vi "GCSTranslator DLL Functions.vi"(0 "System no.":i32=1 min=1 step=1, 1 "Function":T1(ring), 4 "String input":string, 5 "error in":errorcluster, 6 "String buffer":string, 7 "Numerical input":i32, 8 "String input 2":string) -> (14 "DLL I32 Return value":i32, 15 "Boolean output":bool, 16 "String output":string, 17 "Numerical output":i32, 19 "error out":errorcluster)   [LabVIEW 2020]
doc: "This VI calls a given function from GCSTranslator.dll. GCSTranslator.dll must be installed. To call a system-specific function, the system-specific GCS DLL must be installed also. \n\nWarning: For XXX_GcsGetANswer , String buffer must be large enough, otherwise the application may crash. Call XXX_GcsGetANswerSize first to determine necessary string length."
uses:
  Global1.vi
  Global DaisyChain.vi
panel:
  # "This vi calls a given function from GCSTranslator.dll. GCSTranslator.dll must be installed. \nThe system specific GCS DLL must be installed also.\nWARNING: For \"XXXX_GcsGetAnswer\" \"String buffer\" must be large enough, otherwise the \napplication may crash. Call \"XXXX_GcsGetAnswerSize\" first to determine necessary string length."
  # "General inputs:"
  # "Function specific inputs:"
  # "Error handling:"
  # "DLL outputs:"
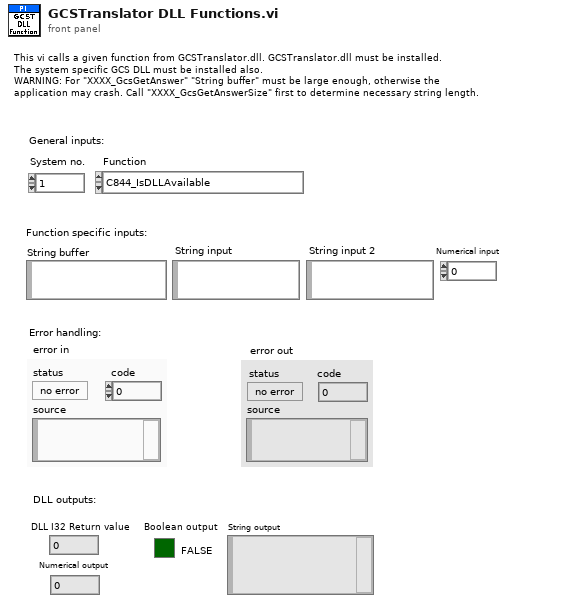
[diagram p1: front panel]
types:
  T1 = enum16{"C844_IsDLLAvailable", "C844_ConnectRS232", "C844_ConnectNIgpib", "C844_IsConnected", "C844_CloseConnection", "C844_GcsCommandset", "C844_GetError", "C844_GcsGetAnswerSize", "C844_GcsGetAnswer", "C843_IsDLLAvailable", "C843_Connect", "C843_IsConnected", "C843_CloseConnection", "C843_GcsCommandset", "C843_GetError", "C843_GcsGetAnswerSize", "C843_GcsGetAnswer", "E710_IsDLLAvailable", "E710_ConnectRS232", "E710_ConnectNIgpib", "E710_IsConnected", "E710_CloseConnection", "E710_GcsCommandset", "E710_GetError", "E710_GcsGetAnswerSize", "E710_GcsGetAnswer", "C843_PM_IsDLLAvailable", "C843_PM_Connect", "C843_PM_IsConnected", "C843_PM_CloseConnection", "C843_PM_GcsCommandset", "C843_PM_GetError", "C843_PM_GcsGetAnswerSize", "C843_PM_GcsGetAnswer", "C843_PM_GetCurrentBoardID", "C843_GetCurrentBoardID", "C865_IsDLLAvailable", "C865_ConnectRS232", "C865_IsConnected", "C865_CloseConnection", "C865_GcsCommandset", "C865_GetError", "C865_GcsGetAnswerSize", "C865_GcsGetAnswer", "C865_GetCurrentInterfaceID", "E761_ConnectPciBoard", "DefineSystem", "CloseConnection", "IsConnected", "ConnectRS232", "ConnectNIgpib", "ConnectPciBoard", "ConnectTCPIP", "GetError", "GcsCommandset", "GCSGetAnswerSize", "GcsGetAnswer", "CloseDaisyChain", "OpenRS232DaisyChain", "ConnectDaisyChainDevice", "ConnectUSB", "ListUSB", "OpenUSBDaisyChain", "OpenTCPIPDaisyChain"}
  T2 = typedef "Available interfaces.ctl" = u16
  T3 = cluster{"RS232 Portnumber":i32, "Timeout":i32, "RS232 Baud rate":u32, "Interface":T2, "GPIB Bus":i32, "GPIB Address":i32, "GPIB Mode":i32}[]
  T4 = cluster{"RS232 Portnumber":i32, "Timeout":i32, "RS232 Baud rate":u32, "Interface":T2, "GPIB Bus":i32, "GPIB Address":i32, "GPIB Mode":i32}
  T5 = typedef "Available DLLs.ctl" = u16
  T6 = typedef "Available DLL interfaces.ctl" = u16
  T7 = cluster{"DLL for Device":T5, "DLL Interface":T6, "Parameter":string}[]
  T8 = cluster{"DLL for Device":T5, "DLL Interface":T6, "Parameter":string}
  T9 = cluster{"No. of devices":i32, "Port ID":i32, "Devices":string[], "Description":string}[]
  T10 = cluster{"No. of devices":i32, "Port ID":i32, "Devices":string[], "Description":string}
  T11 = cluster{"Host address/name":string, "Port":i32, "Board":i32}[]
  T12 = cluster{"Host address/name":string, "Port":i32, "Board":i32}
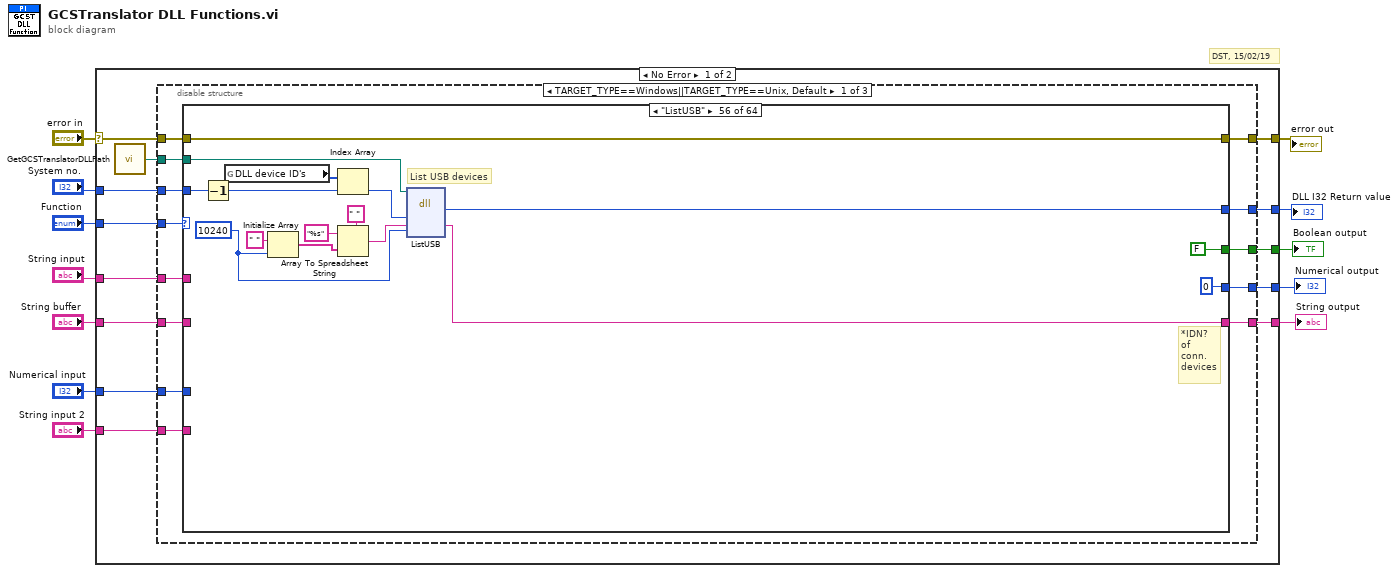
[diagram p0: block diagram]
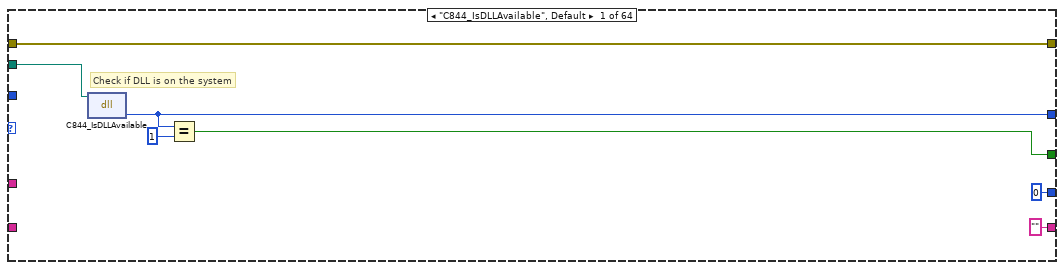
[diagram p2: hidden frame]
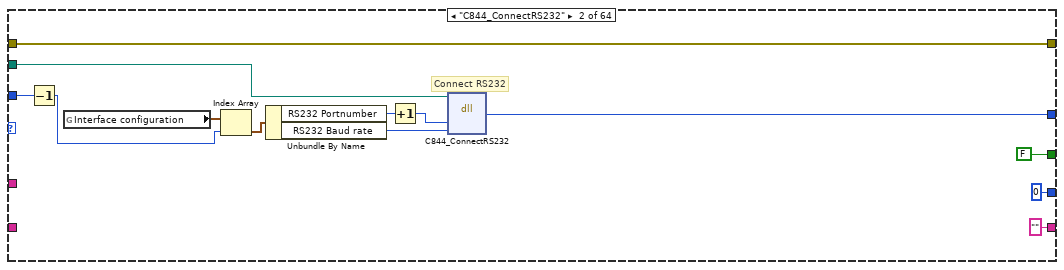
[diagram p3: hidden frame]
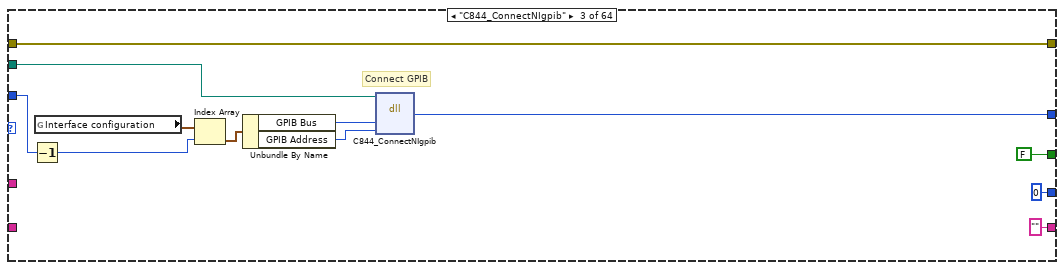
[diagram p4: hidden frame]
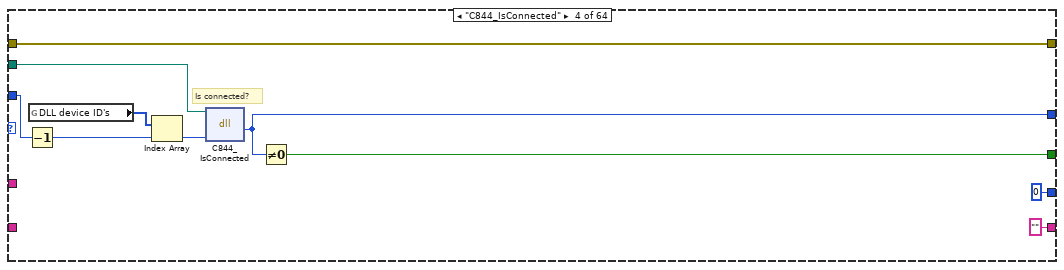
[diagram p5: hidden frame]
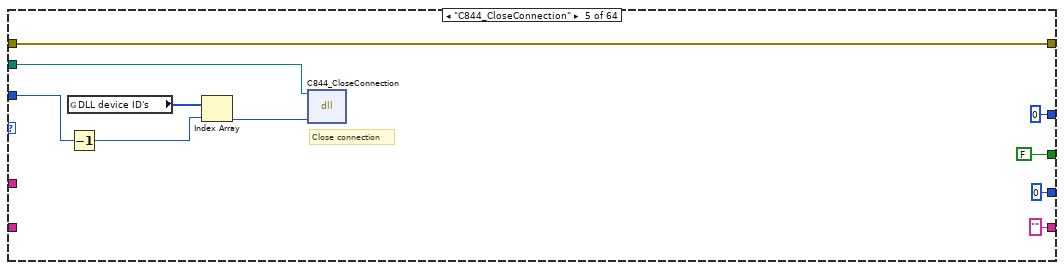
[diagram p6: hidden frame]
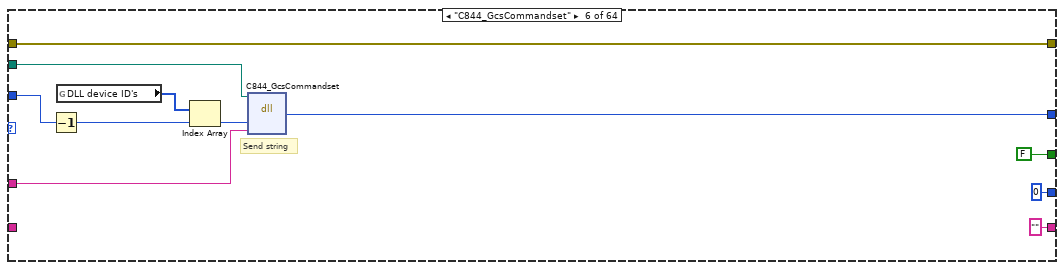
[diagram p7: hidden frame]
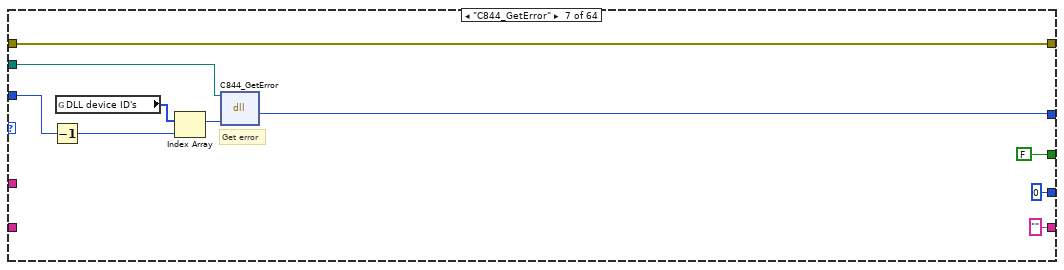
[diagram p8: hidden frame]
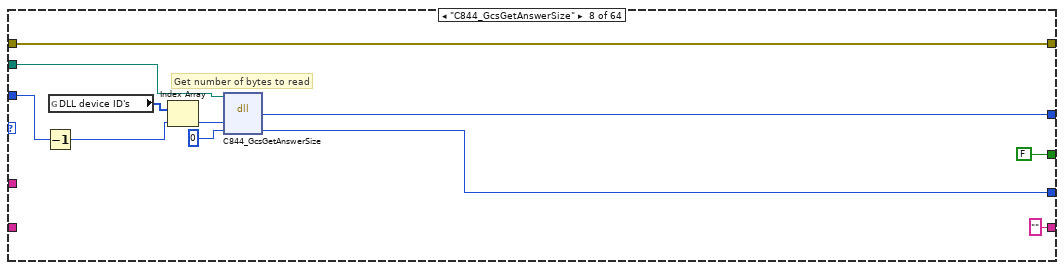
[diagram p9: hidden frame]
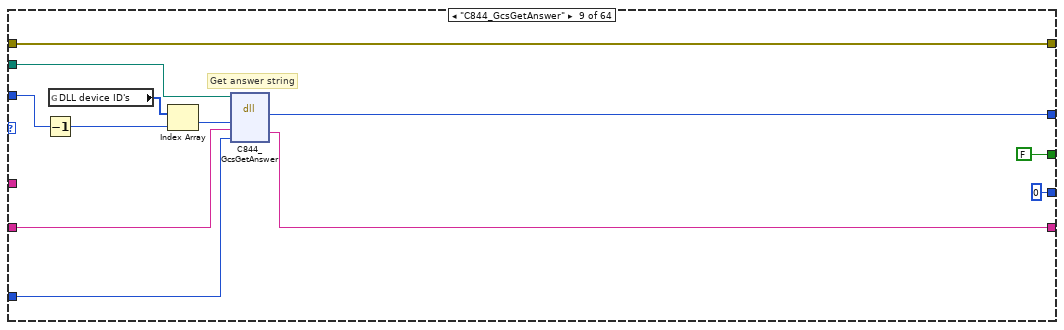
[diagram p10: hidden frame]
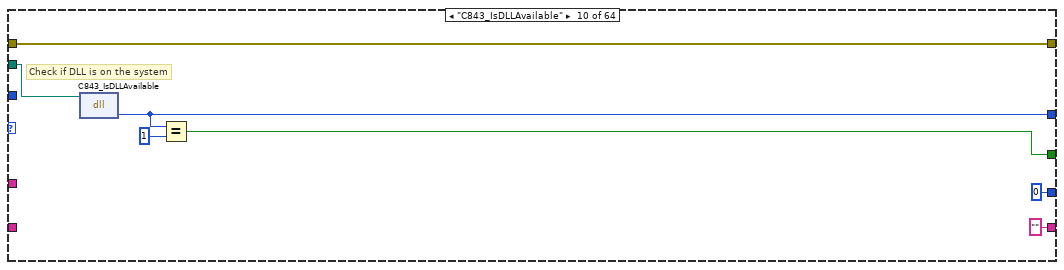
[diagram p11: hidden frame]
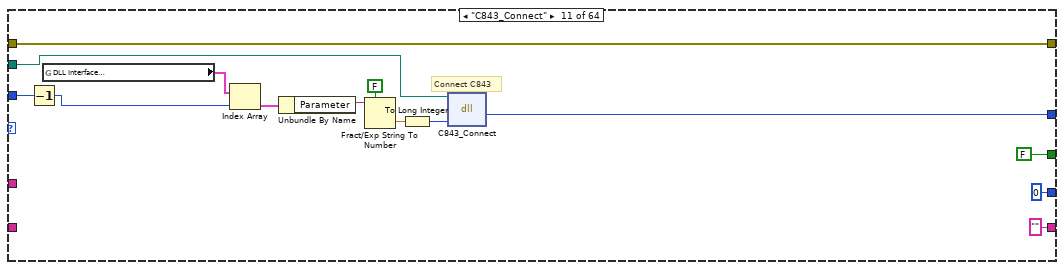
[diagram p12: hidden frame]
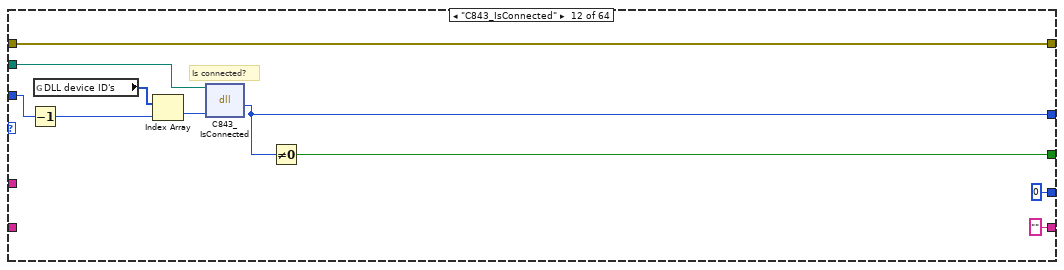
[diagram p13: hidden frame]
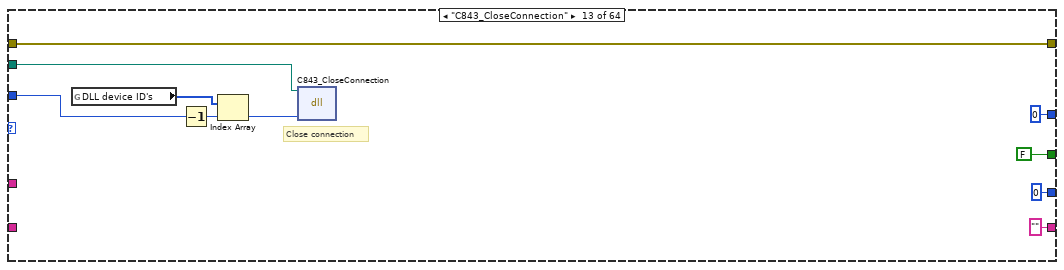
[diagram p14: hidden frame]
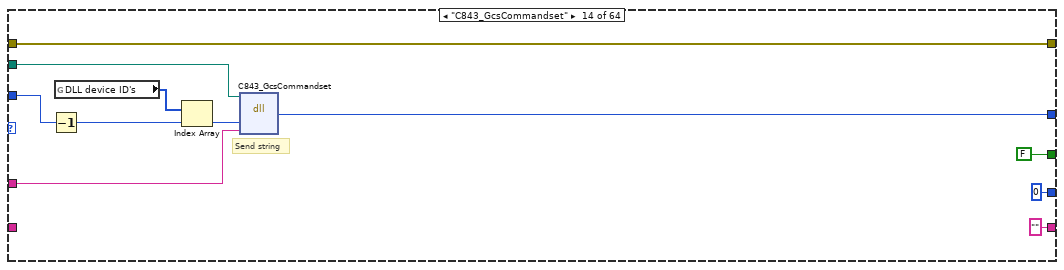
[diagram p15: hidden frame]
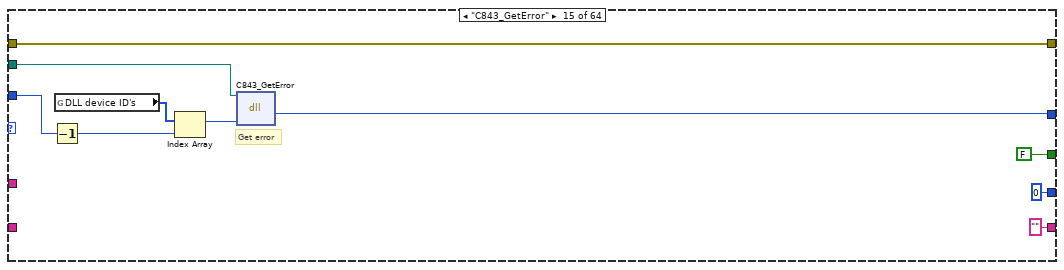
[diagram p16: hidden frame]
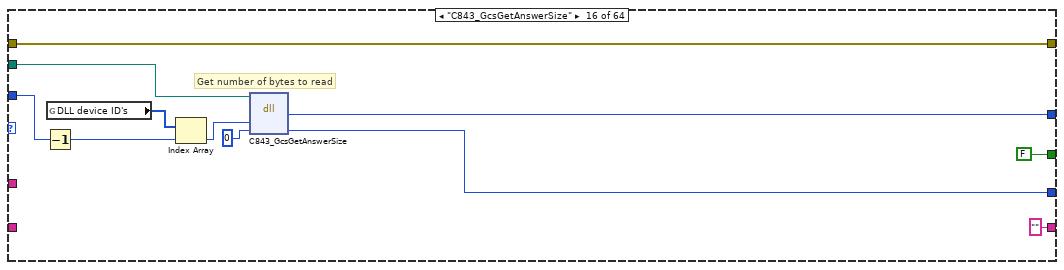
[diagram p17: hidden frame]
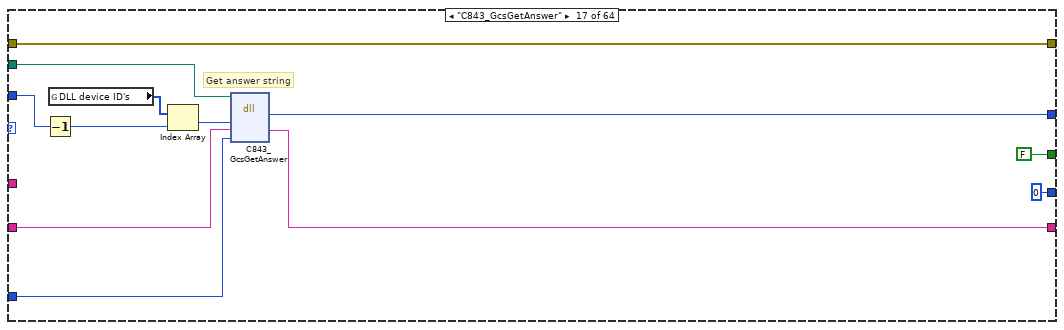
[diagram p18: hidden frame]
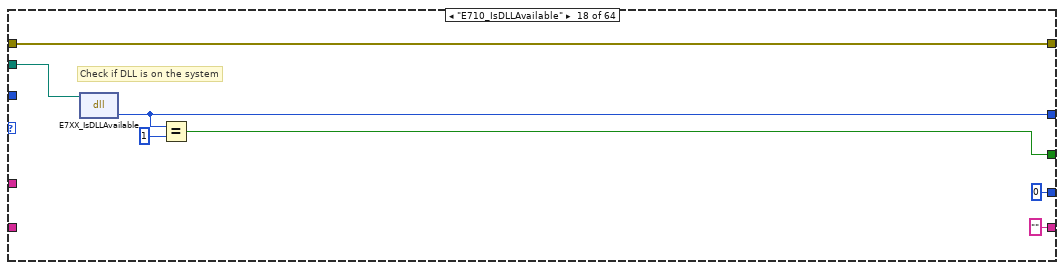
[diagram p19: hidden frame]
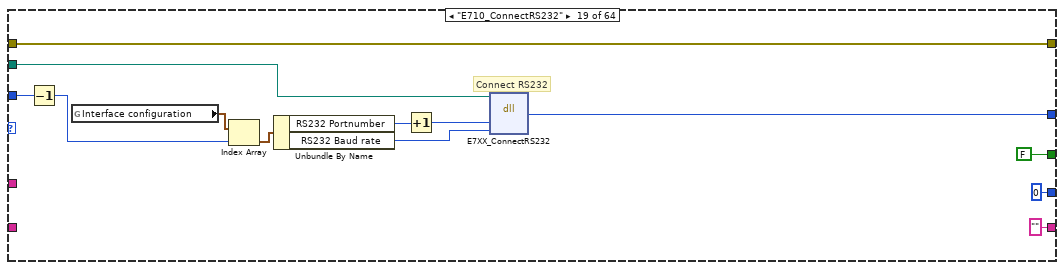
[diagram p20: hidden frame]
diagram:
  # "DST, 15/02/19"
  n1 = case shown="No Error" "error in" {
    selector: "error in" -> [w16 w891]
    tunnel: [w25 w891] -> w12
    tunnel: [w24 0] -> w11
    tunnel: [w23 FALSE] -> w10
    tunnel: "String input" -> [w22 _]
    tunnel: [w21 0 ("iAnswerSize")] -> w8
    tunnel: "String buffer" -> [w20 _]
    tunnel: [w19 "" ("szAnswer")] -> w6
    tunnel: "Numerical input" -> [w18 _]
    tunnel: "String input 2" -> [w17 _]
    tunnel: "System no." -> [w15 _]
    tunnel: "Function" -> [w14 _]
    frame No Error {
      n2 = call "GetGCSTranslatorDLLPath.vi"() -> ("DLL path"=w13:path)  [unwired: 1 in]
      n3 = disable-structure shown="TARGET_TYPE==Windows||TARGET_TYPE==Unix, Default" {
        disable-tunnel: w14 -> [w38 _ _]
        disable-tunnel: w16 -> [w37 w889 w890]
        disable-tunnel: [w36 w889 w890] -> w25
        disable-tunnel: [w35 _ _] -> w24
        disable-tunnel: w15 -> [w34 _ _]
        disable-tunnel: [w33 _ _] -> w23
        disable-tunnel: w22 -> [w32 _ _]
        disable-tunnel: [w31 _ _] -> w21
        disable-tunnel: w20 -> [w30 _ _]
        disable-tunnel: [w29 _ _] -> w19
        disable-tunnel: w18 -> [w28 _ _]
        disable-tunnel: w17 -> [w27 _ _]
        disable-tunnel: w13 -> [w26 _ _]
        frame condition #0 (active) {
          n4 = case shown="\"ListUSB\"" w38 {
            tunnel: w34 -> [_ w52 w65 w75 w85 w96 w106 w116 w129 _ w152 w160 w170 w181 w191 w201 w214 _ w233 w246 w256 w266 w277 w287 w297 w310 _ w334 w341 w351 w362 w372 w382 w395 w411 w425 _ w443 w453 w463 w474 w484 w494 w507 w523 _ w539 w547 w582 w599 w621 w650 w700 w733 w762 w778 w790 w806 w820 w834 w845 w860 w870 w883]
            tunnel: w37 -> [w45 w50 w63 w78 w90 w101 w111 w122 w134 w141 w150 w163 w175 w186 w196 w207 w219 w226 w231 w244 w259 w271 w282 w292 w303 w315 w322 w332 w344 w356 w367 w377 w388 w400 w409 w423 w435 w441 w456 w468 w479 w489 w500 w512 w521 w531 w544 w560 w585 w597 w607 w641 w699 w732 w761 w777 w788 w804 w818 w833 w840 w865 w876 w888]
            tunnel: [w45 w50 w63 w78 w90 w101 w111 w122 w134 w141 w150 w163 w175 w186 w196 w207 w219 w226 w231 w244 w259 w271 w282 w292 w303 w315 w322 w332 w344 w356 w367 w377 w388 w400 w409 w423 w435 w441 w456 w468 w479 w489 w500 w512 w521 w531 w544 w560 w585 w597 w606 w640 w699 w732 w761 w777 w788 w804 w818 w833 w839 w865 w876 w888] -> w36
            tunnel: [w44 w51 w64 w77 0 w100 w110 w120 w133 w140 w151 w162 0 w185 w195 w205 w218 w225 w232 w245 w258 0 w281 w291 w301 w314 w321 w333 w343 0 w366 w376 w386 w399 w410 w424 w434 w442 w455 0 w478 w488 w498 w511 w522 w532 0 0 w584 w598 w620 w649 w676 w715 w750 w768 w789 w805 w819 w827 w838 w864 w874 w887] -> w35
            tunnel: [w42 FALSE FALSE w74 FALSE FALSE FALSE FALSE FALSE w138 FALSE w159 FALSE FALSE FALSE FALSE FALSE w223 FALSE FALSE w255 FALSE FALSE FALSE FALSE FALSE w319 FALSE w340 FALSE FALSE FALSE FALSE FALSE FALSE FALSE w432 FALSE w452 FALSE FALSE FALSE FALSE FALSE FALSE FALSE FALSE FALSE w581 FALSE FALSE FALSE FALSE FALSE FALSE FALSE FALSE FALSE FALSE FALSE FALSE FALSE FALSE FALSE] -> w33
            tunnel: w32 -> [_ _ _ _ _ w94 _ _ _ _ _ _ _ w179 _ _ _ _ _ _ _ _ w275 _ _ _ _ _ _ _ w360 _ _ _ _ _ _ _ _ _ w472 _ _ _ _ w534 _ _ _ _ _ _ _ _ _ _ _ _ _ _ _ w858 _ _]
            tunnel: [0 ("iAnswerSize") 0 ("iAnswerSize") 0 ("iAnswerSize") 0 ("iAnswerSize") 0 ("iAnswerSize") 0 ("iAnswerSize") 0 ("iAnswerSize") w114 0 ("iAnswerSize") 0 ("iAnswerSize") 0 ("iAnswerSize") 0 ("iAnswerSize") 0 ("iAnswerSize") 0 ("iAnswerSize") 0 ("iAnswerSize") w199 0 ("iAnswerSize") 0 ("iAnswerSize") 0 ("iAnswerSize") 0 ("iAnswerSize") 0 ("iAnswerSize") 0 ("iAnswerSize") 0 ("iAnswerSize") 0 ("iAnswerSize") w295 0 ("iAnswerSize") 0 ("iAnswerSize") 0 ("iAnswerSize") 0 ("iAnswerSize") 0 ("iAnswerSize") 0 ("iAnswerSize") 0 ("iAnswerSize") w380 0 ("iAnswerSize") 0 ("iAnswerSize") 0 ("iAnswerSize") 0 ("iAnswerSize") 0 ("iAnswerSize") 0 ("iAnswerSize") 0 ("iAnswerSize") 0 ("iAnswerSize") 0 ("iAnswerSize") w492 0 ("iAnswerSize") 0 ("iAnswerSize") 0 ("iAnswerSize") 0 ("iAnswerSize") 0 ("iAnswerSize") 0 ("iAnswerSize") 0 ("iAnswerSize") 0 ("iAnswerSize") 0 ("iAnswerSize") w675 w714 w747 0 ("iAnswerSize") 0 ("iAnswerSize") 0 ("iAnswerSize") 0 ("iAnswerSize") 0 ("iAnswerSize") 0 ("iAnswerSize") 0 ("iAnswerSize") w868 0 ("iAnswerSize")] -> w31
            tunnel: w30 -> [_ _ _ _ _ _ _ _ w127 _ _ _ _ _ _ _ w212 _ _ _ _ _ _ _ _ w308 _ _ _ _ _ _ _ w393 _ _ _ _ _ _ _ _ _ w505 _ _ _ _ _ _ _ _ _ _ _ _ _ _ _ _ _ _ _ w881]
            tunnel: ["" ("szAnswer") "" ("szAnswer") "" ("szAnswer") "" ("szAnswer") "" ("szAnswer") "" ("szAnswer") "" ("szAnswer") "" ("szAnswer") w126 "" ("szAnswer") "" ("szAnswer") "" ("szAnswer") "" ("szAnswer") "" ("szAnswer") "" ("szAnswer") "" ("szAnswer") w211 "" ("szAnswer") "" ("szAnswer") "" ("szAnswer") "" ("szAnswer") "" ("szAnswer") "" ("szAnswer") "" ("szAnswer") "" ("szAnswer") w307 "" ("szAnswer") "" ("szAnswer") "" ("szAnswer") "" ("szAnswer") "" ("szAnswer") "" ("szAnswer") "" ("szAnswer") w392 "" ("szAnswer") "" ("szAnswer") "" ("szAnswer") "" ("szAnswer") "" ("szAnswer") "" ("szAnswer") "" ("szAnswer") "" ("szAnswer") "" ("szAnswer") w504 "" ("szAnswer") "" ("szAnswer") "" ("szAnswer") "" ("szAnswer") "" ("szAnswer") "" ("szAnswer") "" ("szAnswer") "" ("szAnswer") w674 w713 w745 w766 "" ("szAnswer") "" ("szAnswer") "" ("szAnswer") "" ("szAnswer") "" ("szAnswer") "" ("szAnswer") "" ("szAnswer") w880] -> w29
            tunnel: w28 -> [_ _ _ _ _ _ _ _ w124 _ _ _ _ _ _ _ w209 _ _ _ _ _ _ _ _ w305 _ _ _ _ _ _ _ w390 _ _ _ _ _ _ _ _ _ w502 _ _ _ _ _ _ _ _ _ _ _ _ _ _ _ _ _ _ _ w878]
            tunnel: w27 -> [_ _ _ _ _ _ _ _ _ _ _ _ _ _ _ _ _ _ _ _ _ _ _ _ _ _ _ _ _ _ _ _ _ _ _ _ _ _ _ _ _ _ _ _ _ w533 _ _ _ _ _ _ _ _ _ _ _ _ _ _ _ _ _ _]
            tunnel: w26 -> [w39 w46 w59 w71 w81 w91 w102 w112 w123 w135 w142 w156 w166 w176 w187 w197 w208 w220 w227 w240 w252 w262 w272 w283 w293 w304 w316 w323 w337 w347 w357 w368 w378 w389 w401 w415 w429 w436 w449 w459 w469 w480 w490 w501 w513 w527 w535 w545 w578 w588 w603 w630 w665 w704 w736 w763 w779 w793 w809 w823 w837 w855 w866 w877]
            frame "C844_IsDLLAvailable", Default {
              # "Check if DLL is on the system"
              n5 = dll-call lib="T:/Entwicklung/HostSoftware/LabVIEW/GCSDrivers/source/GCS2LabVIEW/Low Level/GCSTranslator.dll" fn="C844_IsDLLAvailable"(path in=w39) -> ("return type"=w44:i32)  [unwired: 2 in, 2 out]
              n6 = Equal?(x=w44, y=1) -> (x = y?=w42:bool)
            }
            frame "C844_ConnectRS232" {
              # "Connect RS232"
              n7 = Decrement(x=w52) -> (x-1=w54:i32)
              n8 = global read "Global1.vi" "Interface configuration"() -> (w55:T3)
              n9 = Index Array(array=w55, index=w54) -> (element=w53:T4)
              n10 = Unbundle By Name(w53) -> ("RS232 Portnumber"=w56:i32, "RS232 Baud rate"=w58:u32)
              n11 = Increment(x=w56) -> (x+1=w57:i32)
              n12 = dll-call lib="T:/Entwicklung/HostSoftware/LabVIEW/GCSDrivers/source/GCS2LabVIEW/Low Level/GCSTranslator.dll" fn="C844_ConnectRS232"(path in=w46, "nPortNr"=w57, "nBaudRate"=w58) -> ("return type"=w51:i32)  [unwired: 4 in, 2 out]
            }
            frame "C844_ConnectNIgpib" {
              # "Connect GPIB"
              n13 = Decrement(x=w65) -> (x-1=w67:i32)
              n14 = global read "Global1.vi" "Interface configuration"() -> (w68:T3)
              n15 = Index Array(array=w68, index=w67) -> (element=w66:T4)
              n16 = Unbundle By Name(w66) -> ("GPIB Bus"=w70:i32, "GPIB Address"=w69:i32)
              n17 = dll-call lib="T:/Entwicklung/HostSoftware/LabVIEW/GCSDrivers/source/GCS2LabVIEW/Low Level/GCSTranslator.dll" fn="C844_ConnectNIgpib"(path in=w59, "nBoard"=w70, "nDevAddr"=w69) -> ("return type"=w64:i32)  [unwired: 4 in, 2 out]
            }
            frame "C844_IsConnected" {
              # "Is connected?"
              n18 = Decrement(x=w75) -> (x-1=w79:i32)
              n19 = global read "Global1.vi" "DLL device ID's"() -> (w76:i32[])
              n20 = Index Array(array=w76, index=w79) -> (element=w80:i32)
              n21 = dll-call lib="T:/Entwicklung/HostSoftware/LabVIEW/GCSDrivers/source/GCS2LabVIEW/Low Level/GCSTranslator.dll" fn="C844_IsConnected"(path in=w71, "ID"=w80) -> ("return type"=w77:i32)  [unwired: 3 in, 2 out]
              n22 = Not Equal To 0?(x=w77) -> (x != 0?=w74:bool)
            }
            frame "C844_CloseConnection" {
              # "Close connection"
              n23 = global read "Global1.vi" "DLL device ID's"() -> (w87:i32[])
              n24 = Decrement(x=w85) -> (x-1=w88:i32)
              n25 = Index Array(array=w87, index=w88) -> (element=w86:i32)
              n26 = dll-call lib="T:/Entwicklung/HostSoftware/LabVIEW/GCSDrivers/source/GCS2LabVIEW/Low Level/GCSTranslator.dll" fn="C844_CloseConnection"(path in=w81, "ID"=w86) -> ()  [unwired: 3 in, 3 out]
            }
            frame "C844_GcsCommandset" {
              # "Send string"
              n27 = Decrement(x=w96) -> (x-1=w99:i32)
              n28 = global read "Global1.vi" "DLL device ID's"() -> (w98:i32[])
              n29 = Index Array(array=w98, index=w99) -> (element=w97:i32)
              n30 = dll-call lib="T:/Entwicklung/HostSoftware/LabVIEW/GCSDrivers/source/GCS2LabVIEW/Low Level/GCSTranslator.dll" fn="C844_GcsCommandset"(path in=w91, "ID"=w97, "szCommand"=w94) -> ("return type"=w100:i32)  [unwired: 4 in, 2 out]
            }
            frame "C844_GetError" {
              # "Get error"
              n31 = Decrement(x=w106) -> (x-1=w109:i32)
              n32 = global read "Global1.vi" "DLL device ID's"() -> (w108:i32[])
              n33 = Index Array(array=w108, index=w109) -> (element=w107:i32)
              n34 = dll-call lib="T:/Entwicklung/HostSoftware/LabVIEW/GCSDrivers/source/GCS2LabVIEW/Low Level/GCSTranslator.dll" fn="C844_GetError"(path in=w102, "ID"=w107) -> ("return type"=w110:i32)  [unwired: 3 in, 2 out]
            }
            frame "C844_GcsGetAnswerSize" {
              # "Get number of bytes to read"
              n35 = Decrement(x=w116) -> (x-1=w119:i32)
              n36 = global read "Global1.vi" "DLL device ID's"() -> (w118:i32[])
              n37 = Index Array(array=w118, index=w119) -> (element=w117:i32)
              n38 = dll-call lib="T:/Entwicklung/HostSoftware/LabVIEW/GCSDrivers/source/GCS2LabVIEW/Low Level/GCSTranslator.dll" fn="C844_GcsGetAnswerSize"(path in=w112, "ID"=w117, "iAnswerSize"=0) -> ("return type"=w120:i32, "iAnswerSize"=w114:i32)  [unwired: 3 in, 2 out]
            }
            frame "C844_GcsGetAnswer" {
              # "Get answer string"
              n39 = Decrement(x=w129) -> (x-1=w132:i32)
              n40 = global read "Global1.vi" "DLL device ID's"() -> (w131:i32[])
              n41 = Index Array(array=w131, index=w132) -> (element=w130:i32)
              n42 = dll-call lib="T:/Entwicklung/HostSoftware/LabVIEW/GCSDrivers/source/GCS2LabVIEW/Low Level/GCSTranslator.dll" fn="C844_GcsGetAnswer"(path in=w123, "ID"=w130, "szAnswer"=w127, "iAnswerSize"=w124) -> ("return type"=w133:i32, "szAnswer"=w126:string)  [unwired: 4 in, 2 out]
            }
            frame "C843_IsDLLAvailable" {
              # "Check if DLL is on the system"
              n43 = dll-call lib="T:/Entwicklung/HostSoftware/LabVIEW/GCSDrivers/source/GCS2LabVIEW/Low Level/GCSTranslator.dll" fn="C843_IsDLLAvailable"(path in=w135) -> ("return type"=w140:i32)  [unwired: 2 in, 2 out]
              n44 = Equal?(x=w140, y=1) -> (x = y?=w138:bool)
            }
            frame "C843_Connect" {
              # "Connect C843"
              n45 = Decrement(x=w152) -> (x-1=w154:i32)
              n46 = global read "Global1.vi" "DLL Interface\nConfiguration"() -> (w155:T7)
              n47 = Index Array(array=w155, index=w154) -> (element=w153:T8)
              n48 = Unbundle By Name(w153) -> ("Parameter"=w146:string)
              n49 = Fract/Exp String To Number(use system decimal point (T)=FALSE, string=w146) -> (number=w147:dbl)  [unwired: 3 out]
              n50 = To Long Integer(number=w147) -> (32bit integer=w145:i32)
              n51 = dll-call lib="T:/Entwicklung/HostSoftware/LabVIEW/GCSDrivers/source/GCS2LabVIEW/Low Level/GCSTranslator.dll" fn="C843_Connect"(path in=w142, "iBoardNumber"=w145) -> ("return type"=w151:i32)  [unwired: 3 in, 2 out]
            }
            frame "C843_IsConnected" {
              # "Is connected?"
              n52 = Decrement(x=w160) -> (x-1=w164:i32)
              n53 = global read "Global1.vi" "DLL device ID's"() -> (w161:i32[])
              n54 = Index Array(array=w161, index=w164) -> (element=w165:i32)
              n55 = dll-call lib="T:/Entwicklung/HostSoftware/LabVIEW/GCSDrivers/source/GCS2LabVIEW/Low Level/GCSTranslator.dll" fn="C843_IsConnected"(path in=w156, "ID"=w165) -> ("return type"=w162:i32)  [unwired: 3 in, 2 out]
              n56 = Not Equal To 0?(x=w162) -> (x != 0?=w159:bool)
            }
            frame "C843_CloseConnection" {
              # "Close connection"
              n57 = global read "Global1.vi" "DLL device ID's"() -> (w172:i32[])
              n58 = Decrement(x=w170) -> (x-1=w173:i32)
              n59 = Index Array(array=w172, index=w173) -> (element=w171:i32)
              n60 = dll-call lib="T:/Entwicklung/HostSoftware/LabVIEW/GCSDrivers/source/GCS2LabVIEW/Low Level/GCSTranslator.dll" fn="C843_CloseConnection"(path in=w166, "ID"=w171) -> ()  [unwired: 3 in, 3 out]
            }
            frame "C843_GcsCommandset" {
              # "Send string"
              n61 = Decrement(x=w181) -> (x-1=w184:i32)
              n62 = global read "Global1.vi" "DLL device ID's"() -> (w183:i32[])
              n63 = Index Array(array=w183, index=w184) -> (element=w182:i32)
              n64 = dll-call lib="T:/Entwicklung/HostSoftware/LabVIEW/GCSDrivers/source/GCS2LabVIEW/Low Level/GCSTranslator.dll" fn="C843_GcsCommandset"(path in=w176, "ID"=w182, "szCommand"=w179) -> ("return type"=w185:i32)  [unwired: 4 in, 2 out]
            }
            frame "C843_GetError" {
              # "Get error"
              n65 = Decrement(x=w191) -> (x-1=w194:i32)
              n66 = global read "Global1.vi" "DLL device ID's"() -> (w193:i32[])
              n67 = Index Array(array=w193, index=w194) -> (element=w192:i32)
              n68 = dll-call lib="T:/Entwicklung/HostSoftware/LabVIEW/GCSDrivers/source/GCS2LabVIEW/Low Level/GCSTranslator.dll" fn="C843_GetError"(path in=w187, "ID"=w192) -> ("return type"=w195:i32)  [unwired: 3 in, 2 out]
            }
            frame "C843_GcsGetAnswerSize" {
              # "Get number of bytes to read"
              n69 = Decrement(x=w201) -> (x-1=w204:i32)
              n70 = global read "Global1.vi" "DLL device ID's"() -> (w203:i32[])
              n71 = Index Array(array=w203, index=w204) -> (element=w202:i32)
              n72 = dll-call lib="T:/Entwicklung/HostSoftware/LabVIEW/GCSDrivers/source/GCS2LabVIEW/Low Level/GCSTranslator.dll" fn="C843_GcsGetAnswerSize"(path in=w197, "ID"=w202, "iAnswerSize"=0) -> ("return type"=w205:i32, "iAnswerSize"=w199:i32)  [unwired: 3 in, 2 out]
            }
            frame "C843_GcsGetAnswer" {
              # "Get answer string"
              n73 = Decrement(x=w214) -> (x-1=w217:i32)
              n74 = global read "Global1.vi" "DLL device ID's"() -> (w216:i32[])
              n75 = Index Array(array=w216, index=w217) -> (element=w215:i32)
              n76 = dll-call lib="T:/Entwicklung/HostSoftware/LabVIEW/GCSDrivers/source/GCS2LabVIEW/Low Level/GCSTranslator.dll" fn="C843_GcsGetAnswer"(path in=w208, "ID"=w215, "szAnswer"=w212, "iAnswerSize"=w209) -> ("return type"=w218:i32, "szAnswer"=w211:string)  [unwired: 4 in, 2 out]
            }
            frame "E710_IsDLLAvailable" {
              # "Check if DLL is on the system"
              n77 = dll-call lib="T:/Entwicklung/HostSoftware/LabVIEW/GCSDrivers/source/GCS2LabVIEW/Low Level/GCSTranslator.dll" fn="E7XX_IsDLLAvailable"(path in=w220) -> ("return type"=w225:i32)  [unwired: 2 in, 2 out]
              n78 = Equal?(x=w225, y=1) -> (x = y?=w223:bool)
            }
            frame "E710_ConnectRS232" {
              # "Connect RS232"
              n79 = Decrement(x=w233) -> (x-1=w235:i32)
              n80 = global read "Global1.vi" "Interface configuration"() -> (w236:T3)
              n81 = Index Array(array=w236, index=w235) -> (element=w234:T4)
              n82 = Unbundle By Name(w234) -> ("RS232 Portnumber"=w237:i32, "RS232 Baud rate"=w239:u32)
              n83 = Increment(x=w237) -> (x+1=w238:i32)
              n84 = dll-call lib="T:/Entwicklung/HostSoftware/LabVIEW/GCSDrivers/source/GCS2LabVIEW/Low Level/GCSTranslator.dll" fn="E7XX_ConnectRS232"(path in=w227, "nPortNr"=w238, "nBaudRate"=w239) -> ("return type"=w232:i32)  [unwired: 4 in, 2 out]
            }
            frame "E710_ConnectNIgpib" {
              # "Connect GPIB"
              n85 = Decrement(x=w246) -> (x-1=w248:i32)
              n86 = global read "Global1.vi" "Interface configuration"() -> (w249:T3)
              n87 = Index Array(array=w249, index=w248) -> (element=w247:T4)
              n88 = Unbundle By Name(w247) -> ("GPIB Bus"=w251:i32, "GPIB Address"=w250:i32)
              n89 = dll-call lib="T:/Entwicklung/HostSoftware/LabVIEW/GCSDrivers/source/GCS2LabVIEW/Low Level/GCSTranslator.dll" fn="E7XX_ConnectNIgpib"(path in=w240, "nBoard"=w251, "nDevAddr"=w250) -> ("return type"=w245:i32)  [unwired: 4 in, 2 out]
            }
            frame "E710_IsConnected" {
              # "Is connected?"
              n90 = global read "Global1.vi" "DLL device ID's"() -> (w257:i32[])
              n91 = Decrement(x=w256) -> (x-1=w260:i32)
              n92 = Index Array(array=w257, index=w260) -> (element=w261:i32)
              n93 = dll-call lib="T:/Entwicklung/HostSoftware/LabVIEW/GCSDrivers/source/GCS2LabVIEW/Low Level/GCSTranslator.dll" fn="E7XX_IsConnected"(path in=w252, "ID"=w261) -> ("return type"=w258:i32)  [unwired: 3 in, 2 out]
              n94 = Not Equal To 0?(x=w258) -> (x != 0?=w255:bool)
            }
            frame "E710_CloseConnection" {
              # "Close connection"
              n95 = global read "Global1.vi" "DLL device ID's"() -> (w268:i32[])
              n96 = Decrement(x=w266) -> (x-1=w269:i32)
              n97 = Index Array(array=w268, index=w269) -> (element=w267:i32)
              n98 = dll-call lib="T:/Entwicklung/HostSoftware/LabVIEW/GCSDrivers/source/GCS2LabVIEW/Low Level/GCSTranslator.dll" fn="E7XX_CloseConnection"(path in=w262, "ID"=w267) -> ()  [unwired: 3 in, 3 out]
            }
            frame "E710_GcsCommandset" {
              # "Send string"
              n99 = global read "Global1.vi" "DLL device ID's"() -> (w279:i32[])
              n100 = Decrement(x=w277) -> (x-1=w280:i32)
              n101 = Index Array(array=w279, index=w280) -> (element=w278:i32)
              n102 = dll-call lib="T:/Entwicklung/HostSoftware/LabVIEW/GCSDrivers/source/GCS2LabVIEW/Low Level/GCSTranslator.dll" fn="E7XX_GcsCommandset"(path in=w272, "ID"=w278, "szCommand"=w275) -> ("return type"=w281:i32)  [unwired: 4 in, 2 out]
            }
            frame "E710_GetError" {
              # "Get error"
              n103 = Decrement(x=w287) -> (x-1=w290:i32)
              n104 = global read "Global1.vi" "DLL device ID's"() -> (w289:i32[])
              n105 = Index Array(array=w289, index=w290) -> (element=w288:i32)
              n106 = dll-call lib="T:/Entwicklung/HostSoftware/LabVIEW/GCSDrivers/source/GCS2LabVIEW/Low Level/GCSTranslator.dll" fn="E7XX_GetError"(path in=w283, "ID"=w288) -> ("return type"=w291:i32)  [unwired: 3 in, 2 out]
            }
            frame "E710_GcsGetAnswerSize" {
              # "Get number of bytes to read"
              n107 = Decrement(x=w297) -> (x-1=w300:i32)
              n108 = global read "Global1.vi" "DLL device ID's"() -> (w299:i32[])
              n109 = Index Array(array=w299, index=w300) -> (element=w298:i32)
              n110 = dll-call lib="T:/Entwicklung/HostSoftware/LabVIEW/GCSDrivers/source/GCS2LabVIEW/Low Level/GCSTranslator.dll" fn="E7XX_GcsGetAnswerSize"(path in=w293, "ID"=w298, "iAnswerSize"=0) -> ("return type"=w301:i32, "iAnswerSize"=w295:i32)  [unwired: 3 in, 2 out]
            }
            frame "E710_GcsGetAnswer" {
              # "Get answer string"
              n111 = Decrement(x=w310) -> (x-1=w313:i32)
              n112 = global read "Global1.vi" "DLL device ID's"() -> (w312:i32[])
              n113 = Index Array(array=w312, index=w313) -> (element=w311:i32)
              n114 = dll-call lib="T:/Entwicklung/HostSoftware/LabVIEW/GCSDrivers/source/GCS2LabVIEW/Low Level/GCSTranslator.dll" fn="E7XX_GcsGetAnswer"(path in=w304, "ID"=w311, "szAnswer"=w308, "iAnswerSize"=w305) -> ("return type"=w314:i32, "szAnswer"=w307:string)  [unwired: 4 in, 2 out]
            }
            frame "C843_PM_IsDLLAvailable" {
              # "Check if DLL is on the system"
              n115 = dll-call lib="T:/Entwicklung/HostSoftware/LabVIEW/GCSDrivers/source/GCS2LabVIEW/Low Level/GCSTranslator.dll" fn="C843_PM_IsDLLAvailable"(path in=w316) -> ("return type"=w321:i32)  [unwired: 2 in, 2 out]
              n116 = Equal?(x=w321, y=1) -> (x = y?=w319:bool)
            }
            frame "C843_PM_Connect" {
              # "Connect C843_PM"
              n117 = Decrement(x=w334) -> (x-1=w324:i32)
              n118 = global read "Global1.vi" "DLL Interface\nConfiguration"() -> (w336:T7)
              n119 = Index Array(array=w336, index=w324) -> (element=w335:T8)
              n120 = Unbundle By Name(w335) -> ("Parameter"=w328:string)
              n121 = Fract/Exp String To Number(use system decimal point (T)=FALSE, string=w328) -> (number=w329:dbl)  [unwired: 3 out]
              n122 = To Long Integer(number=w329) -> (32bit integer=w327:i32)
              n123 = dll-call lib="T:/Entwicklung/HostSoftware/LabVIEW/GCSDrivers/source/GCS2LabVIEW/Low Level/GCSTranslator.dll" fn="C843_PM_Connect"(path in=w323, "iBoardNumber"=w327) -> ("return type"=w333:i32)  [unwired: 3 in, 2 out]
            }
            frame "C843_PM_IsConnected" {
              # "Is connected?"
              n124 = Decrement(x=w341) -> (x-1=w345:i32)
              n125 = global read "Global1.vi" "DLL device ID's"() -> (w342:i32[])
              n126 = Index Array(array=w342, index=w345) -> (element=w346:i32)
              n127 = dll-call lib="T:/Entwicklung/HostSoftware/LabVIEW/GCSDrivers/source/GCS2LabVIEW/Low Level/GCSTranslator.dll" fn="C843_PM_IsConnected"(path in=w337, "ID"=w346) -> ("return type"=w343:i32)  [unwired: 3 in, 2 out]
              n128 = Not Equal To 0?(x=w343) -> (x != 0?=w340:bool)
            }
            frame "C843_PM_CloseConnection" {
              # "Close connection"
              n129 = Decrement(x=w351) -> (x-1=w354:i32)
              n130 = global read "Global1.vi" "DLL device ID's"() -> (w353:i32[])
              n131 = Index Array(array=w353, index=w354) -> (element=w352:i32)
              n132 = dll-call lib="T:/Entwicklung/HostSoftware/LabVIEW/GCSDrivers/source/GCS2LabVIEW/Low Level/GCSTranslator.dll" fn="C843_PM_CloseConnection"(path in=w347, "ID"=w352) -> ()  [unwired: 3 in, 3 out]
            }
            frame "C843_PM_GcsCommandset" {
              # "Send string"
              n133 = Decrement(x=w362) -> (x-1=w365:i32)
              n134 = global read "Global1.vi" "DLL device ID's"() -> (w364:i32[])
              n135 = Index Array(array=w364, index=w365) -> (element=w363:i32)
              n136 = dll-call lib="T:/Entwicklung/HostSoftware/LabVIEW/GCSDrivers/source/GCS2LabVIEW/Low Level/GCSTranslator.dll" fn="C843_PM_GcsCommandset"(path in=w357, "ID"=w363, "szCommand"=w360) -> ("return type"=w366:i32)  [unwired: 4 in, 2 out]
            }
            frame "C843_PM_GetError" {
              # "Get error"
              n137 = Decrement(x=w372) -> (x-1=w375:i32)
              n138 = global read "Global1.vi" "DLL device ID's"() -> (w374:i32[])
              n139 = Index Array(array=w374, index=w375) -> (element=w373:i32)
              n140 = dll-call lib="T:/Entwicklung/HostSoftware/LabVIEW/GCSDrivers/source/GCS2LabVIEW/Low Level/GCSTranslator.dll" fn="C843_PM_GetError"(path in=w368, "ID"=w373) -> ("return type"=w376:i32)  [unwired: 3 in, 2 out]
            }
            frame "C843_PM_GcsGetAnswerSize" {
              # "Get number of bytes to read"
              n141 = Decrement(x=w382) -> (x-1=w385:i32)
              n142 = global read "Global1.vi" "DLL device ID's"() -> (w384:i32[])
              n143 = Index Array(array=w384, index=w385) -> (element=w383:i32)
              n144 = dll-call lib="T:/Entwicklung/HostSoftware/LabVIEW/GCSDrivers/source/GCS2LabVIEW/Low Level/GCSTranslator.dll" fn="C843_PM_GcsGetAnswerSize"(path in=w378, "ID"=w383, "iAnswerSize"=0) -> ("return type"=w386:i32, "iAnswerSize"=w380:i32)  [unwired: 3 in, 2 out]
            }
            frame "C843_PM_GcsGetAnswer" {
              # "Get answer string"
              n145 = Decrement(x=w395) -> (x-1=w398:i32)
              n146 = global read "Global1.vi" "DLL device ID's"() -> (w397:i32[])
              n147 = Index Array(array=w397, index=w398) -> (element=w396:i32)
              n148 = dll-call lib="T:/Entwicklung/HostSoftware/LabVIEW/GCSDrivers/source/GCS2LabVIEW/Low Level/GCSTranslator.dll" fn="C843_PM_GcsGetAnswer"(path in=w389, "ID"=w396, "szAnswer"=w393, "iAnswerSize"=w390) -> ("return type"=w399:i32, "szAnswer"=w392:string)  [unwired: 4 in, 2 out]
            }
            frame "C843_PM_GetCurrentBoardID" {
              # "Get current ID C843_PM"
              n149 = Decrement(x=w411) -> (x-1=w413:i32)
              n150 = global read "Global1.vi" "DLL Interface\nConfiguration"() -> (w414:T7)
              n151 = Index Array(array=w414, index=w413) -> (element=w412:T8)
              n152 = Unbundle By Name(w412) -> ("Parameter"=w405:string)
              n153 = Fract/Exp String To Number(use system decimal point (T)=FALSE, string=w405) -> (number=w406:dbl)  [unwired: 3 out]
              n154 = To Long Integer(number=w406) -> (32bit integer=w404:i32)
              n155 = dll-call lib="T:/Entwicklung/HostSoftware/LabVIEW/GCSDrivers/source/GCS2LabVIEW/Low Level/GCSTranslator.dll" fn="C843_PM_GetCurrentBoardId"(path in=w401, "iBoardNumber"=w404) -> ("return type"=w410:i32)  [unwired: 3 in, 2 out]
            }
            frame "C843_GetCurrentBoardID" {
              # "Get current ID C843"
              n156 = Decrement(x=w425) -> (x-1=w427:i32)
              n157 = global read "Global1.vi" "DLL Interface\nConfiguration"() -> (w428:T7)
              n158 = Index Array(array=w428, index=w427) -> (element=w426:T8)
              n159 = Unbundle By Name(w426) -> ("Parameter"=w419:string)
              n160 = Fract/Exp String To Number(use system decimal point (T)=FALSE, string=w419) -> (number=w420:dbl)  [unwired: 3 out]
              n161 = To Long Integer(number=w420) -> (32bit integer=w418:i32)
              n162 = dll-call lib="T:/Entwicklung/HostSoftware/LabVIEW/GCSDrivers/source/GCS2LabVIEW/Low Level/GCSTranslator.dll" fn="C843_GetCurrentBoardId"(path in=w415, "iBoardNumber"=w418) -> ("return type"=w424:i32)  [unwired: 3 in, 2 out]
            }
            frame "C865_IsDLLAvailable" {
              # "Check if DLL is on the system"
              n163 = dll-call lib="T:/Entwicklung/HostSoftware/LabVIEW/GCSDrivers/source/GCS2LabVIEW/Low Level/GCSTranslator.dll" fn="C865_IsDLLAvailable"(path in=w429) -> ("return type"=w434:i32)  [unwired: 2 in, 2 out]
              n164 = Equal?(x=w434, y=1) -> (x = y?=w432:bool)
            }
            frame "C865_ConnectRS232" {
              # "Connect RS232"
              n165 = Decrement(x=w443) -> (x-1=w437:i32)
              n166 = global read "Global1.vi" "Interface configuration"() -> (w445:T3)
              n167 = Index Array(array=w445, index=w437) -> (element=w444:T4)
              n168 = Unbundle By Name(w444) -> ("RS232 Portnumber"=w446:i32, "RS232 Baud rate"=w448:u32)
              n169 = Increment(x=w446) -> (x+1=w447:i32)
              n170 = dll-call lib="T:/Entwicklung/HostSoftware/LabVIEW/GCSDrivers/source/GCS2LabVIEW/Low Level/GCSTranslator.dll" fn="C865_ConnectRS232"(path in=w436, "nPortNr"=w447, "nBaudRate"=w448) -> ("return type"=w442:i32)  [unwired: 4 in, 2 out]
            }
            frame "C865_IsConnected" {
              # "Is connected?"
              n171 = global read "Global1.vi" "DLL device ID's"() -> (w454:i32[])
              n172 = Decrement(x=w453) -> (x-1=w457:i32)
              n173 = Index Array(array=w454, index=w457) -> (element=w458:i32)
              n174 = dll-call lib="T:/Entwicklung/HostSoftware/LabVIEW/GCSDrivers/source/GCS2LabVIEW/Low Level/GCSTranslator.dll" fn="C865_IsConnected"(path in=w449, "ID"=w458) -> ("return type"=w455:i32)  [unwired: 3 in, 2 out]
              n175 = Not Equal To 0?(x=w455) -> (x != 0?=w452:bool)
            }
            frame "C865_CloseConnection" {
              # "Close connection"
              n176 = global read "Global1.vi" "DLL device ID's"() -> (w465:i32[])
              n177 = Decrement(x=w463) -> (x-1=w466:i32)
              n178 = Index Array(array=w465, index=w466) -> (element=w464:i32)
              n179 = dll-call lib="T:/Entwicklung/HostSoftware/LabVIEW/GCSDrivers/source/GCS2LabVIEW/Low Level/GCSTranslator.dll" fn="C865_CloseConnection"(path in=w459, "ID"=w464) -> ()  [unwired: 3 in, 3 out]
            }
            frame "C865_GcsCommandset" {
              # "Send string"
              n180 = global read "Global1.vi" "DLL device ID's"() -> (w476:i32[])
              n181 = Decrement(x=w474) -> (x-1=w477:i32)
              n182 = Index Array(array=w476, index=w477) -> (element=w475:i32)
              n183 = dll-call lib="T:/Entwicklung/HostSoftware/LabVIEW/GCSDrivers/source/GCS2LabVIEW/Low Level/GCSTranslator.dll" fn="C865_GcsCommandset"(path in=w469, "ID"=w475, "szCommand"=w472) -> ("return type"=w478:i32)  [unwired: 4 in, 2 out]
            }
            frame "C865_GetError" {
              # "Get error"
              n184 = Decrement(x=w484) -> (x-1=w487:i32)
              n185 = global read "Global1.vi" "DLL device ID's"() -> (w486:i32[])
              n186 = Index Array(array=w486, index=w487) -> (element=w485:i32)
              n187 = dll-call lib="T:/Entwicklung/HostSoftware/LabVIEW/GCSDrivers/source/GCS2LabVIEW/Low Level/GCSTranslator.dll" fn="C865_GetError"(path in=w480, "ID"=w485) -> ("return type"=w488:i32)  [unwired: 3 in, 2 out]
            }
            frame "C865_GcsGetAnswerSize" {
              # "Get number of bytes to read"
              n188 = global read "Global1.vi" "DLL device ID's"() -> (w496:i32[])
              n189 = Decrement(x=w494) -> (x-1=w497:i32)
              n190 = Index Array(array=w496, index=w497) -> (element=w495:i32)
              n191 = dll-call lib="T:/Entwicklung/HostSoftware/LabVIEW/GCSDrivers/source/GCS2LabVIEW/Low Level/GCSTranslator.dll" fn="C865_GcsGetAnswerSize"(path in=w490, "ID"=w495, "iAnswerSize"=0) -> ("return type"=w498:i32, "iAnswerSize"=w492:i32)  [unwired: 3 in, 2 out]
            }
            frame "C865_GcsGetAnswer" {
              # "Get answer string"
              n192 = Decrement(x=w507) -> (x-1=w510:i32)
              n193 = global read "Global1.vi" "DLL device ID's"() -> (w509:i32[])
              n194 = Index Array(array=w509, index=w510) -> (element=w508:i32)
              n195 = dll-call lib="T:/Entwicklung/HostSoftware/LabVIEW/GCSDrivers/source/GCS2LabVIEW/Low Level/GCSTranslator.dll" fn="C865_GcsGetAnswer"(path in=w501, "ID"=w508, "szAnswer"=w505, "iAnswerSize"=w502) -> ("return type"=w511:i32, "szAnswer"=w504:string)  [unwired: 4 in, 2 out]
            }
            frame "C865_GetCurrentInterfaceID" {
              # "Get current ID C865"
              n196 = Decrement(x=w523) -> (x-1=w525:i32)
              n197 = global read "Global1.vi" "DLL Interface\nConfiguration"() -> (w526:T7)
              n198 = Index Array(array=w526, index=w525) -> (element=w524:T8)
              n199 = Unbundle By Name(w524) -> ("Parameter"=w517:string)
              n200 = Fract/Exp String To Number(use system decimal point (T)=FALSE, string=w517) -> (number=w518:dbl)  [unwired: 3 out]
              n201 = To Long Integer(number=w518) -> (32bit integer=w516:i32)
              n202 = dll-call lib="T:/Entwicklung/HostSoftware/LabVIEW/GCSDrivers/source/GCS2LabVIEW/Low Level/GCSTranslator.dll" fn="C865_GetCurrentInterfaceId"(path in=w513, "iBoardNumber"=w516) -> ("return type"=w522:i32)  [unwired: 3 in, 2 out]
            }
            frame "DefineSystem" {
              # "Define which GCS dll to use and for which system"
              n203 = dll-call lib="T:/Entwicklung/HostSoftware/LabVIEW/GCSDrivers/source/GCS2LabVIEW/Low Level/GCSTranslator.dll" fn="DefineSystem"(path in=w527, "szDLLName"=w534, "szCtrlPrefix"=w533) -> ("return type"=w532:i32)  [unwired: 4 in, 2 out]
            }
            frame "CloseConnection" {
              # "Close connection"
              n204 = global read "Global1.vi" "DLL device ID's"() -> (w541:i32[])
              n205 = Decrement(x=w539) -> (x-1=w542:i32)
              n206 = Index Array(array=w541, index=w542) -> (element=w540:i32)
              n207 = dll-call lib="T:/Entwicklung/HostSoftware/LabVIEW/GCSDrivers/source/GCS2LabVIEW/Low Level/GCSTranslator.dll" fn="CloseConnection"(path in=w535, "ID"=w540) -> ()  [unwired: 3 in, 3 out]
            }
            frame "CloseDaisyChain" {
              # "CloseDaisyChain"
              n208 = Decrement(x=w547) -> (x-1=w552:i32)
              n209 = global read "Global1.vi" "DLL device ID's"() -> (w558:i32[])
              n210 = global read "Global DaisyChain.vi" "DaisyChain configuration"() -> (w550:T9)
              n211 = global read "Global1.vi" "Number of\nsystems"() -> (w548:i32)
              n212 = Index Array(array=w558, index=w552) -> (element=w557:i32)
              n213 = Max & Min(x=w547, y=w548) -> (max(x,y)=w546:i32)  [unwired: 1 out]
              n214 = Index Array(array=w550, index=w552) -> (element=w553:T10)
              n215 = Unbundle By Name(w553) -> ("Port ID"=w551:i32)
              n216 = for {
                N: w546 -> [_]
                tunnel: w550 -> [w566]
                shift-right: [w568] -> w549
                shift-left: w550 -> [w567]
                tunnel: w551 -> [w564]
                i -> [w562]
                n217 = Index Array(array=w566, index=w562) -> (element=w561:T10)
                n218 = Unbundle By Name(w561) -> ("Port ID"=w565:i32)
                n219 = Equal?(x=w565, y=w564) -> (x = y?=w563:bool)
                n220 = case shown="True" w563 {
                  tunnel: [w569 w574] -> w568
                  tunnel: w567 -> [w569 w572]
                  tunnel: w562 -> [_ w573]
                  tunnel: w561 -> [_ w571]
                  frame False {
                  }
                  frame True {
                    n221 = Bundle By Name(cluster=w571, "Port ID"=-1, "No. of devices"=0, "Devices"=string[] []) -> (w570:T10)
                    n222 = Replace Array Subset(array=w572, new element=w570, index=w573) -> (w574:T9)
                  }
                }
              }
              n223 = dll-call lib="T:/Entwicklung/HostSoftware/LabVIEW/GCSDrivers/source/GCS2LabVIEW/Low Level/GCSTranslator.dll" fn="CloseDaisyChain"(path in=w545, "ID"=w557, "iPortID"=w551) -> ()  [unwired: 4 in, 3 out]
              n224 = global write "Global DaisyChain.vi" "DaisyChain configuration"(w549) -> ()
            }
            frame "IsConnected" {
              # "Is connected?"
              n225 = global read "Global1.vi" "DLL device ID's"() -> (w583:i32[])
              n226 = Decrement(x=w582) -> (x-1=w586:i32)
              n227 = Index Array(array=w583, index=w586) -> (element=w587:i32)
              n228 = dll-call lib="T:/Entwicklung/HostSoftware/LabVIEW/GCSDrivers/source/GCS2LabVIEW/Low Level/GCSTranslator.dll" fn="IsConnected"(path in=w578, "ID"=w587) -> ("return type"=w584:i32)  [unwired: 3 in, 2 out]
              n229 = Not Equal To 0?(x=w584) -> (x != 0?=w581:bool)
            }
            frame "ConnectRS232" {
              # "Port ID"
              # "Connect RS232"
              n230 = Decrement(x=w599) -> (x-1=w590:i32)
              n231 = global read "Global1.vi" "DLL device ID's"() -> (w591:i32[])
              n232 = global read "Global1.vi" "Interface configuration"() -> (w601:T3)
              n233 = Index Array(array=w591, index=w590) -> (element=w589:i32)
              n234 = Index Array(array=w601, index=w590) -> (element=w600:T4)
              n235 = Unbundle By Name(w600) -> ("RS232 Portnumber"=w602:i32, "RS232 Baud rate"=w593:u32)
              n236 = Increment(x=w602) -> (x+1=w592:i32)
              n237 = dll-call lib="T:/Entwicklung/HostSoftware/LabVIEW/GCSDrivers/source/GCS2LabVIEW/Low Level/GCSTranslator.dll" fn="ConnectRS232"(path in=w588, "ID"=w589, "nPortNr"=w592, "nBaudRate"=w593) -> ("return type"=w598:i32)  [unwired: 5 in, 2 out]
            }
            frame "ConnectDaisyChainDevice" {
              # "Connect DaisyChainDevice"
              n238 = Decrement(x=w621) -> (x-1=w610:i32)
              n239 = global read "Global1.vi" "DLL device ID's"() -> (w616:i32[])
              n240 = global read "Global DaisyChain.vi" "DaisyChain configuration"() -> (w614:T9)
              n241 = Index Array(array=w616, index=w610) -> (element=w615:i32)
              n242 = Index Array(array=w614, index=w610) -> (element=w613:T10)
              n243 = Unbundle By Name(w613) -> ("Port ID"=w609:i32, "Description"=w604:string)
              n244 = Fract/Exp String To Number(use system decimal point (T)=FALSE, string=w604) -> (number=w611:dbl)  [unwired: 3 out]
              n245 = Less Than 0?(x=w609) -> (x < 0?=w605:bool)
              n246 = To Long Integer(number=w611) -> (32bit integer=w608:i32)
              n247 = case shown="False" w605 {
                tunnel: [w627 -1] -> w620
                tunnel: w615 -> [w626 _]
                tunnel: w608 -> [w625 _]
                tunnel: w609 -> [w624 _]
                tunnel: [w623 errorcluster {"status"=TRUE, "code"=100, "source"="Check DeviceID, cable\nconnections and\nbaudrate settings."} ("error in")] -> w606
                tunnel: w607 -> [w623 _]
                tunnel: w603 -> [w622 _]
                frame False {
                  n248 = dll-call lib="T:/Entwicklung/HostSoftware/LabVIEW/GCSDrivers/source/GCS2LabVIEW/Low Level/GCSTranslator.dll" fn="ConnectDaisyChainDevice"(path in=w622, "ID"=w626, "iPortId"=w624, "iDeviceNumber"=w625) -> ("return type"=w627:i32)  [unwired: 5 in, 2 out]
                }
                frame True {
                }
              }
            }
            frame "ConnectUSB" {
              # "ConnectUSB"
              n249 = Decrement(x=w650) -> (x-1=w634:i32)
              n250 = global read "Global1.vi" "DLL device ID's"() -> (w645:i32[])
              n251 = global read "Global1.vi" "DLL Interface\nConfiguration"() -> (w643:T7)
              n252 = global read "Global DaisyChain.vi" "DaisyChain configuration"() -> (w633:T9)
              n253 = Index Array(array=w645, index=w634) -> (element=w644:i32)
              n254 = Index Array(array=w643, index=w634) -> (element=w642:T8)
              n255 = Index Array(array=w633, index=w634) -> (element=w632:T10)
              n256 = Unbundle By Name(w642) -> ("Parameter"=w636:string, "DLL Interface"=w637:T6)
              n257 = Unbundle By Name(w632) -> ("Description"=w631:string)
              n258 = case shown="1" w637 {
                tunnel: [w651 w652 w653 w654 w655 w656 w657] -> w635
                tunnel: w636 -> [w651 w652 w653 w654 w655 w656 _]
                tunnel: w631 -> [_ _ _ _ _ _ w657]
                frame 0, Default {
                }
                frame 1 {
                }
                frame 2 {
                }
                frame 3 {
                }
                frame 4 {
                }
                frame 5 {
                }
                frame 6 {
                }
              }
              n259 = Not Equal?(x=w635, y="") -> (x != y?=w638:bool)
              n260 = case shown="True" w638 {
                tunnel: [-1 w664] -> w649
                tunnel: w644 -> [_ w663]
                tunnel: [errorcluster {"status"=TRUE, "code"=100, "source"="ConnectUSB: \nNo Serial Number given."} ("error in") w662] -> w640
                tunnel: w641 -> [_ w662]
                tunnel: w635 -> [_ w661]
                tunnel: w630 -> [_ w660]
                frame False {
                }
                frame True {
                  n261 = dll-call lib="T:/Entwicklung/HostSoftware/LabVIEW/GCSDrivers/source/GCS2LabVIEW/Low Level/GCSTranslator.dll" fn="ConnectUSB"(path in=w660, "ID"=w663, "szDescription"=w661) -> ("return type"=w664:i32)  [unwired: 4 in, 2 out]
                }
              }
            }
            frame "OpenRS232DaisyChain" {
              w678 = i16 0 ("width (-)")
              w690 = 12700 ("dimension size")
              # "*IDN?\nof\nconn.\ndevices"
              # "Nr. of\ndevices"
              # "OpenRS232DaisyChain"
              n262 = Decrement(x=w700) -> (x-1=w666:i32)
              n263 = global read "Global1.vi" "Interface configuration"() -> (w702:T3)
              n264 = global read "Global1.vi" "DLL device ID's"() -> (w697:i32[])
              n265 = Divide(x=w690, y=2) -> (x/y=w683:dbl)
              n266 = To Long Integer(number=w683) -> (32bit integer=w691:i32)
              n267 = Initialize Array(" ", w691) -> (w694:string[])
              n268 = Index Array(array=w702, index=w666) -> (element=w701:T4)
              n269 = Index Array(array=w697, index=w666) -> (element=w696:i32)
              n270 = Unbundle By Name(w701) -> ("RS232 Portnumber"=w703:i32, "RS232 Baud rate"=w679:u32)
              n271 = Array To Spreadsheet String(delimiter (Tab)=" ", array=w694, 3:"%s" ("format string")) -> (spreadsheet string=w688:string)
              n272 = Increment(x=w703) -> (x+1=w682:i32)
              n273 = global read "Global1.vi" "DLL Interface\nConfiguration"() -> (w671:T7)
              n274 = dll-call lib="T:/Entwicklung/HostSoftware/LabVIEW/GCSDrivers/source/GCS2LabVIEW/Low Level/GCSTranslator.dll" fn="OpenRS232DaisyChain"(path in=w665, "ID"=w696, "iPortNumber"=w682, "iBaudRate"=w679, "szBuffer"=w688, "maxlen"=w690) -> ("return type"=w676:i32, "pNrDev"=w675:i32, "szBuffer"=w674:string)  [unwired: 6 in, 3 out]
              n275 = Number To Decimal String(number=w682, width (-)=w678) -> (decimal integer string=w681:string)
              n276 = Number To Decimal String(number=w679, width (-)=w678) -> (decimal integer string=w677:string)
              n277 = call "Get lines from string.vi"("Input string"=w674) -> ("Strings"=w673:string[])  [unwired: 2 in, 16 out]
              n278 = global read "Global DaisyChain.vi" "DaisyChain configuration"() -> (w667:T9)
              n279 = Concatenate Strings("COM" ("string"), w681, "::" ("string"), w677) -> (w669:string)
              n280 = Index Array(array=w671, index=w666) -> (element=w672:T8)
              n281 = Bundle By Name(cluster=w672, "Parameter"=w669) -> (w670:T8)
              n282 = Replace Array Subset(array=w671, new element=w670, index=w666) -> (w668:T7)
              n283 = Index Array(array=w667, index=w666) -> (element=w687:T10)
              n284 = Bundle By Name(cluster=w687, "Port ID"=w676, "No. of devices"=w675, "Devices"=w673) -> (w685:T10)
              n285 = global write "Global1.vi" "DLL Interface\nConfiguration"(w668) -> ()
              n286 = Replace Array Subset(array=w667, new element=w685, index=w666) -> (w686:T9)
              n287 = global write "Global DaisyChain.vi" "DaisyChain configuration"(w686) -> ()
            }
            frame "OpenTCPIPDaisyChain" {
              w723 = 12700 ("dimension size")
              # "*IDN?\nof\nconn.\ndevices"
              # "Nr. of\ndevices"
              # "OpenTCPIPDaisyChain"
              n288 = Decrement(x=w733) -> (x-1=w705:i32)
              n289 = global read "Global1.vi" "DLL device ID's"() -> (w730:i32[])
              n290 = global read "Global1.vi" "TCP/IP Configuration"() -> (w735:T11)
              n291 = Divide(x=w723, y=2) -> (x/y=w716:dbl)
              n292 = To Long Integer(number=w716) -> (32bit integer=w724:i32)
              n293 = Initialize Array(" ", w724) -> (w727:string[])
              n294 = Index Array(array=w730, index=w705) -> (element=w729:i32)
              n295 = Index Array(array=w735, index=w705) -> (element=w734:T12)
              n296 = Array To Spreadsheet String(delimiter (Tab)=" ", array=w727, 3:"%s" ("format string")) -> (spreadsheet string=w721:string)
              n297 = Unbundle By Name(w734) -> ("Host address/name"=w710:string, "Port"=w711:i32)
              n298 = dll-call lib="T:/Entwicklung/HostSoftware/LabVIEW/GCSDrivers/source/GCS2LabVIEW/Low Level/GCSTranslator.dll" fn="OpenTCPIPDaisyChain"(path in=w704, "ID"=w729, "szHostname"=w710, "port"=w711, "szDeviceIDNs"=w721, "iBufferSize"=w723) -> ("return type"=w715:i32, "pNumberOfConnectedDaisyChainDevices"=w714:i32, "szDeviceIDNs"=w713:string)  [unwired: 5 in, 4 out]
              n299 = call "Get lines from string.vi"("Input string"=w713) -> ("Strings"=w712:string[])  [unwired: 2 in, 16 out]
              n300 = global read "Global DaisyChain.vi" "DaisyChain configuration"() -> (w719:T9)
              n301 = global read "Global1.vi" "DLL Interface\nConfiguration"() -> (w708:T7)
              n302 = Index Array(array=w719, index=w705) -> (element=w720:T10)
              n303 = Bundle By Name(cluster=w720, "Port ID"=w715, "No. of devices"=w714, "Devices"=w712) -> (w717:T10)
              n304 = Index Array(array=w708, index=w705) -> (element=w709:T8)
              n305 = Bundle By Name(cluster=w709, "Parameter"=w710) -> (w707:T8)
              n306 = Replace Array Subset(array=w708, new element=w707, index=w705) -> (w706:T7)
              n307 = Replace Array Subset(array=w719, new element=w717, index=w705) -> (w718:T9)
              n308 = global write "Global1.vi" "DLL Interface\nConfiguration"(w706) -> ()
              n309 = global write "Global DaisyChain.vi" "DaisyChain configuration"(w718) -> ()
            }
            frame "OpenUSBDaisyChain" {
              w746 = 12700 ("dimension size")
              # "*IDN?\nof\nconn.\ndevices"
              # "Nr. of\ndevices"
              # "OpenUSBDaisyChain"
              n310 = Decrement(x=w762) -> (x-1=w737:i32)
              n311 = global read "Global1.vi" "DLL Interface\nConfiguration"() -> (w742:T7)
              n312 = global read "Global1.vi" "DLL device ID's"() -> (w760:i32[])
              n313 = Index Array(array=w760, index=w737) -> (element=w759:i32)
              n314 = Divide(x=w746, y=2) -> (x/y=w751:dbl)
              n315 = To Long Integer(number=w751) -> (32bit integer=w754:i32)
              n316 = Index Array(array=w742, index=w737) -> (element=w741:T8)
              n317 = Initialize Array(" ", w754) -> (w757:string[])
              n318 = Unbundle By Name(w741) -> ("Parameter"=w740:string)
              n319 = Array To Spreadsheet String(delimiter (Tab)=" ", array=w757, 3:"%s" ("format string")) -> (spreadsheet string=w748:string)
              n320 = dll-call lib="T:/Entwicklung/HostSoftware/LabVIEW/GCSDrivers/source/GCS2LabVIEW/Low Level/GCSTranslator.dll" fn="OpenUSBDaisyChain"(path in=w736, "ID"=w759, "SN"=w740, "szBuffer"=w748, "maxlen"=w746) -> ("return type"=w750:i32, "pNrDev"=w747:i32, "szBuffer"=w745:string)  [unwired: 4 in, 4 out]
              n321 = call "Get lines from string.vi"("Input string"=w745) -> ("Strings"=w749:string[])  [unwired: 2 in, 16 out]
              n322 = global read "Global DaisyChain.vi" "DaisyChain configuration"() -> (w738:T9)
              n323 = Index Array(array=w738, index=w737) -> (element=w743:T10)
              n324 = Bundle By Name(cluster=w743, "Port ID"=w750, "No. of devices"=w747, "Devices"=w749) -> (w752:T10)
              n325 = Replace Array Subset(array=w738, new element=w752, index=w737) -> (w739:T9)
              n326 = global write "Global DaisyChain.vi" "DaisyChain configuration"(w739) -> ()
            }
            frame "ListUSB" {
              w764 = 10240 ("dimension size")
              # "*IDN?\nof\nconn.\ndevices"
              # "List USB devices"
              n327 = Decrement(x=w778) -> (x-1=w769:i32)
              n328 = global read "Global1.vi" "DLL device ID's"() -> (w775:i32[])
              n329 = Initialize Array(" ", w764) -> (w772:string[])
              n330 = Index Array(array=w775, index=w769) -> (element=w774:i32)
              n331 = Array To Spreadsheet String(delimiter (Tab)=" ", array=w772, 3:"%s" ("format string")) -> (spreadsheet string=w767:string)
              n332 = dll-call lib="T:/Entwicklung/HostSoftware/LabVIEW/GCSDrivers/source/GCS2LabVIEW/Low Level/GCSTranslator.dll" fn="ListUSB"(path in=w763, "ID"=w774, "szDescriptionList"=w767, "maxlen"=w764) -> ("return type"=w768:i32, "szDescriptionList"=w766:string)  [unwired: 4 in, 2 out]
            }
            frame "ConnectNIgpib" {
              # "Connect GPIB"
              n333 = global read "Global1.vi" "DLL device ID's"() -> (w780:i32[])
              n334 = global read "Global1.vi" "Interface configuration"() -> (w792:T3)
              n335 = Decrement(x=w790) -> (x-1=w782:i32)
              n336 = Index Array(array=w780, index=w782) -> (element=w781:i32)
              n337 = Index Array(array=w792, index=w782) -> (element=w791:T4)
              n338 = Unbundle By Name(w791) -> ("GPIB Bus"=w783:i32, "GPIB Address"=w784:i32)
              n339 = dll-call lib="T:/Entwicklung/HostSoftware/LabVIEW/GCSDrivers/source/GCS2LabVIEW/Low Level/GCSTranslator.dll" fn="ConnectNIgpib"(path in=w779, "ID"=w781, "nBoard"=w783, "nDevAddr"=w784) -> ("return type"=w789:i32)  [unwired: 5 in, 2 out]
            }
            frame "ConnectPciBoard" {
              # "Connect"
              n340 = Decrement(x=w806) -> (x-1=w794:i32)
              n341 = global read "Global1.vi" "DLL Interface\nConfiguration"() -> (w808:T7)
              n342 = global read "Global1.vi" "DLL device ID's"() -> (w797:i32[])
              n343 = Index Array(array=w797, index=w794) -> (element=w795:i32)
              n344 = Index Array(array=w808, index=w794) -> (element=w807:T8)
              n345 = Unbundle By Name(w807) -> ("Parameter"=w800:string)
              n346 = Fract/Exp String To Number(use system decimal point (T)=FALSE, string=w800) -> (number=w801:dbl)  [unwired: 3 out]
              n347 = To Long Integer(number=w801) -> (32bit integer=w796:i32)
              n348 = dll-call lib="T:/Entwicklung/HostSoftware/LabVIEW/GCSDrivers/source/GCS2LabVIEW/Low Level/GCSTranslator.dll" fn="ConnectPciBoard"(path in=w793, "ID"=w795, "iBoardNumber"=w796) -> ("return type"=w805:i32)  [unwired: 4 in, 2 out]
            }
            frame "E761_ConnectPciBoard" {
              # "E761 Connect"
              n349 = Decrement(x=w820) -> (x-1=w811:i32)
              n350 = global read "Global1.vi" "DLL Interface\nConfiguration"() -> (w822:T7)
              n351 = Index Array(array=w822, index=w811) -> (element=w821:T8)
              n352 = Unbundle By Name(w821) -> ("Parameter"=w814:string)
              n353 = Fract/Exp String To Number(use system decimal point (T)=FALSE, string=w814) -> (number=w815:dbl)  [unwired: 3 out]
              n354 = To Long Integer(number=w815) -> (32bit integer=w810:i32)
              n355 = dll-call lib="T:/Entwicklung/HostSoftware/LabVIEW/GCSDrivers/source/GCS2LabVIEW/Low Level/GCSTranslator.dll" fn="E7XX_ConnectPciBoard"(path in=w809, "IBoardNumber"=w810) -> ("return type"=w819:i32)  [unwired: 3 in, 2 out]
            }
            frame "ConnectTCPIP" {
              # "Connect TCP-IP"
              n356 = Decrement(x=w834) -> (x-1=w828:i32)
              n357 = global read "Global1.vi" "TCP/IP Configuration"() -> (w836:T11)
              n358 = global read "Global1.vi" "DLL device ID's"() -> (w829:i32[])
              n359 = Index Array(array=w836, index=w828) -> (element=w835:T12)
              n360 = Index Array(array=w829, index=w828) -> (element=w826:i32)
              n361 = Unbundle By Name(w835) -> ("Host address/name"=w825:string, "Port"=w824:i32)
              n362 = dll-call lib="T:/Entwicklung/HostSoftware/LabVIEW/GCSDrivers/source/GCS2LabVIEW/Low Level/GCSTranslator.dll" fn="ConnectTCPIP"(path in=w823, "ID"=w826, "szHostname"=w825, "port"=w824) -> ("return type"=w827:i32)  [unwired: 4 in, 3 out]
            }
            frame "GetError" {
              # "Get error"
              n363 = Decrement(x=w845) -> (x-1=w848:i32)
              n364 = global read "Global1.vi" "DLL device ID's"() -> (w847:i32[])
              n365 = Index Array(array=w847, index=w848) -> (element=w846:i32)
              n366 = dll-call lib="T:/Entwicklung/HostSoftware/LabVIEW/GCSDrivers/source/GCS2LabVIEW/Low Level/GCSTranslator.dll" fn="GetError"(path in=w837, "ID"=w846) -> ("return type"=w838:i32)  [unwired: 3 in, 2 out]
              n367 = Not Equal To 0?(x=w838) -> (x != 0?=w841:bool)
              n368 = case shown="True" w841 {
                tunnel: w840 -> [w849 w853]
                tunnel: [w849 w854] -> w839
                tunnel: w838 -> [_ w851]
                frame False {
                }
                frame True {
                  n369 = Bundle By Name(cluster=w853, "status"=TRUE, "code"=w851, "source"="GCSTranslator DLL Functions.vi: \nDLL reports error.") -> (w854:errorcluster)
                }
              }
            }
            frame "GcsCommandset" {
              # "Send string"
              n370 = Decrement(x=w860) -> (x-1=w863:i32)
              n371 = global read "Global1.vi" "DLL device ID's"() -> (w862:i32[])
              n372 = Index Array(array=w862, index=w863) -> (element=w861:i32)
              n373 = dll-call lib="T:/Entwicklung/HostSoftware/LabVIEW/GCSDrivers/source/GCS2LabVIEW/Low Level/GCSTranslator.dll" fn="GcsCommandset"(path in=w855, "ID"=w861, "szCommand"=w858) -> ("return type"=w864:i32)  [unwired: 4 in, 2 out]
            }
            frame "GCSGetAnswerSize" {
              # "Get number of bytes to read"
              n374 = Decrement(x=w870) -> (x-1=w873:i32)
              n375 = global read "Global1.vi" "DLL device ID's"() -> (w872:i32[])
              n376 = Index Array(array=w872, index=w873) -> (element=w871:i32)
              n377 = dll-call lib="T:/Entwicklung/HostSoftware/LabVIEW/GCSDrivers/source/GCS2LabVIEW/Low Level/GCSTranslator.dll" fn="GcsGetAnswerSize"(path in=w866, "ID"=w871, "iAnswerSize"=0) -> ("return type"=w874:i32, "iAnswerSize"=w868:i32)  [unwired: 3 in, 2 out]
            }
            frame "GcsGetAnswer" {
              # "Get answer string"
              n378 = Decrement(x=w883) -> (x-1=w886:i32)
              n379 = global read "Global1.vi" "DLL device ID's"() -> (w885:i32[])
              n380 = Index Array(array=w885, index=w886) -> (element=w884:i32)
              n381 = dll-call lib="T:/Entwicklung/HostSoftware/LabVIEW/GCSDrivers/source/GCS2LabVIEW/Low Level/GCSTranslator.dll" fn="GcsGetAnswer"(path in=w877, "ID"=w884, "szAnswer"=w881, "iAnswerSize"=w878) -> ("return type"=w887:i32, "szAnswer"=w880:string)  [unwired: 4 in, 2 out]
            }
          }
        }
        frame condition #1 {
        }
        frame condition #2 {
        }
      }
    }
    frame Error {
    }
  }
  "error out" <- w12
  "DLL I32 Return value" <- w11
  "Boolean output" <- w10
  "Numerical output" <- w8
  "String output" <- w6
